vi "LogError.vi"(0 "Error To Log":errorcluster, 2 "Context (\"Error\")":string="Error", 4 "reference in":refnum<class "MLA.lvclass">, 5 "Stop?":bool) -> (1 "Cleaned Error":errorcluster, 3 "Stop?":bool, 7 "reference out":refnum<class "MLA.lvclass">)   [LabVIEW 2023, in "MLA.lvclass"]
uses:
  MLA.lvclass
  S5Tools/ErrorLog/ErrorLog.lvclass
panel:
  out "Error String":string
  out "error out":errorcluster
  in  "error in (no error)":errorcluster
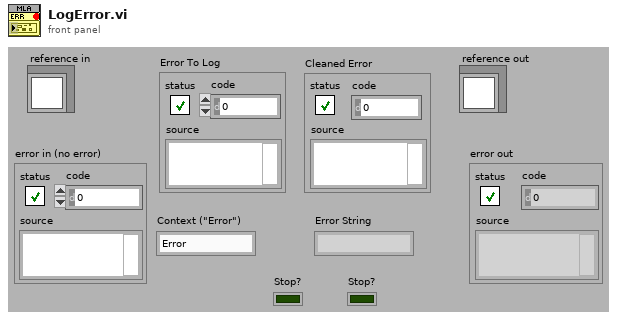
[diagram p1: front panel]
types:
  T1 = typedef "MLA.lvclass/ObjectAttributes.ctl" = cluster{"App Name":string, "App Version":string, "Revision History":string, "Log File Path":path, "Config INI File":path, "Config Path":path, "Log Archive Path":path, "Msg Q's":refnum<queue>[], "VI":refnum<vi>, "ErrLog":refnum<class "ErrorLog.lvclass">}
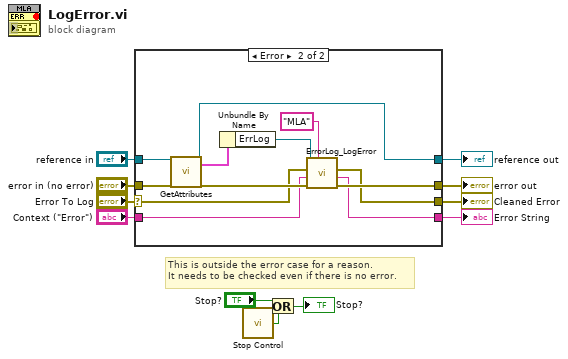
[diagram p0: block diagram]
diagram:
  # "This is outside the error case for a reason.\nIt needs to be checked even if there is no error."
  n1 = case shown="Error" "Error To Log" {
    selector: "Error To Log" -> [w13 w19]
    tunnel: [w13 w21] -> w11
    tunnel: [w12 w15] -> w9
    tunnel: "reference in" -> [w12 w25]
    tunnel: "error in (no error)" -> [_ w24]
    tunnel: "Context (\"Error\")" -> [_ w17]
    tunnel: [_ w18] -> w5
    tunnel: [_ w16] -> w4
    frame No Error {
    }
    frame Error {
      n2 = call "GetAttributes.vi"("MLA"=w25, "error in (no error)"=w24) -> ("MLA"=w15:refnum<class "MLA.lvclass">, "Data"=w23:T1, "error out"=w22:errorcluster)  [unwired: 14 in, 1 out]
      n3 = Unbundle By Name(w23) -> ("ErrLog"=w20:refnum<class "ErrorLog.lvclass">)
      n4 = call-dynamic "ErrorLog_LogError.vi"("Owner (\"Error\")"="MLA" ("Owner (\"Error\")"), "error in (no error)"=w22, "Context (\"Error\")"=w17, "Error To Log"=w19, "reference in"=w20) -> ("error out"=w21:errorcluster, "Error String"=w16:string, "Cleaned Error"=w18:errorcluster)  [unwired: 2 in, 2 out]
    }
  }
  "error out" <- w11
  "reference out" <- w9
  "Cleaned Error" <- w5
  "Error String" <- w4
  n5 = call "Stop Control.vi"() -> ("Stop?"=w3:bool)  [unwired: 1 in]
  n6 = Or(x="Stop?", y=w3) -> (x .or. y?=→"Stop?":bool)
